vi "Dequeue Message.vi"(8 "Error In":errorcluster, 11 "Message Queue":refnum<queue>) -> (0 "Error Out":errorcluster, 1 "Message Data":variant, 2 "Message":string, 3 "dup Message Queue":refnum<queue>)   [LabVIEW 2017]
uses:
  Desktop/Semestr 8/LabVIEW Advanced/LabVIEW Core 3/Exercises/LabVIEW Core 3/Course Project/support/Message Queue/Message Cluster.ctl
  Desktop/Semestr 8/LabVIEW Advanced/LabVIEW Core 3/Exercises/LabVIEW Core 3/Course Project/support/Message Queue/Message Queue.lvlib
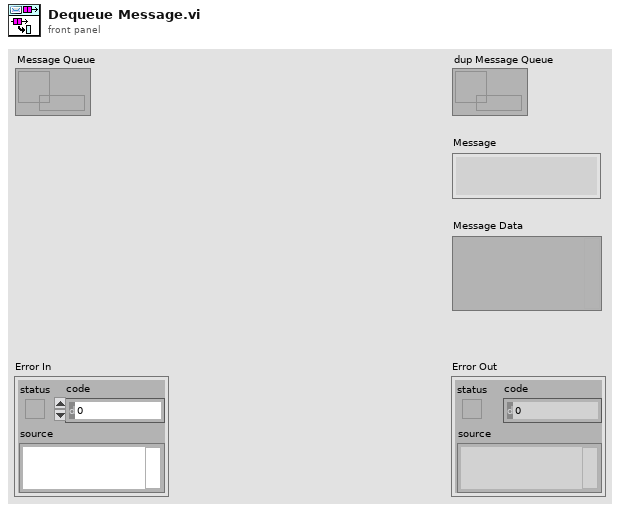
[diagram p1: front panel]
types:
  T1 = typedef "Message Queue.lvlib/Message Cluster.ctl" = cluster{"Message":string, "Message Data":variant}
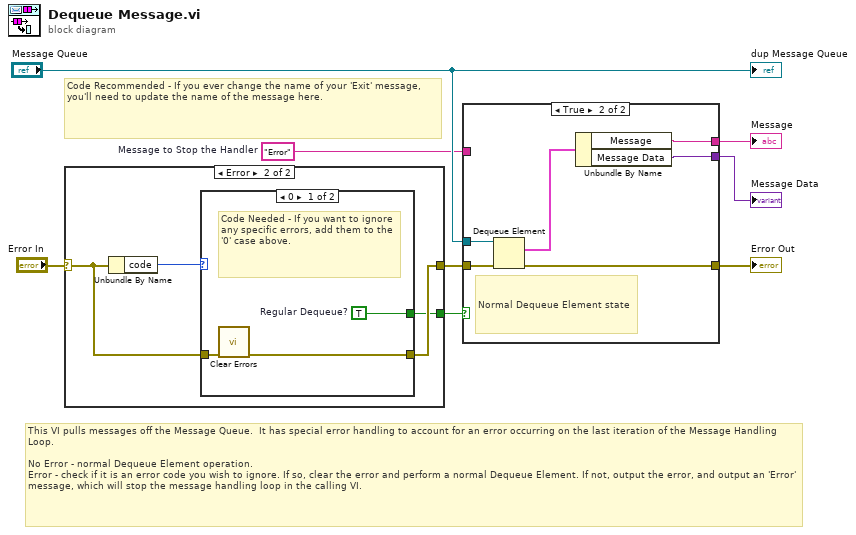
[diagram p0: block diagram]
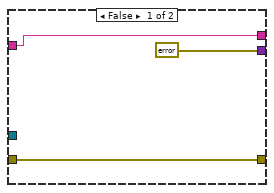
[diagram p2: hidden frame]
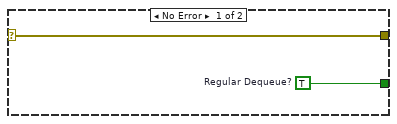
[diagram p3: hidden frame]
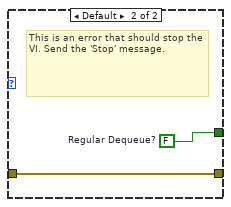
[diagram p4: hidden frame]
diagram:
  w1 = "Error"  # Message to Stop the Handler
  # "Code Recommended - If you ever change the name of your 'Exit' message, you'll need to update the name of the message here."
  # "This VI pulls messages off the Message Queue.  It has special error handling to account for an error occurring on the last iteration of the Message Handling Loop.\n\nNo Error - normal Dequeue Element operation.\nError - check if it is an error code you wish to ignore. If so, clear the error and perform a normal Dequeue Element. If not, output the error, and output an 'Error' message, which will stop the message handling loop in the calling VI."
  n1 = case shown="Error" "Error In" {
    selector: "Error In" -> [w10 w13]
    tunnel: [w10 w12] -> w6
    tunnel: [w9 w11] -> w5
    frame No Error {
      w9 = TRUE  # Regular Dequeue?
    }
    frame Error {
      n2 = Unbundle By Name(w13) -> ("code"=w14:i32)
      n3 = case shown="0" w14 {
        tunnel: [w17 w19] -> w12
        tunnel: w13 -> [w16 w19]
        tunnel: [w15 w18] -> w11
        frame 0 {
          w15 = TRUE  # Regular Dequeue?
          # "Code Needed - If you want to ignore any specific errors, add them to the '0' case above."
          n4 = call <vilib>:"Clear Errors.vi"("error in (no error)"=w16) -> ("error out"=w17:errorcluster)  [unwired: 5 in, 1 out]
        }
        frame Default {
          w18 = FALSE  # Regular Dequeue?
          # "This is an error that should stop the VI. Send the 'Stop' message."
        }
      }
    }
  }
  n5 = case shown="True" w5 {
    tunnel: [w22 w28] -> w7
    tunnel: w6 -> [w22 w27]
    tunnel: "Message Queue" -> [_ w26]
    tunnel: [w21 w24] -> w3
    tunnel: [errorcluster {"status"=FALSE, "code"=0, "source"=""} ("error IO") w23] -> w2
    tunnel: w1 -> [w21 _]
    frame False {
    }
    frame True {
      # "Normal Dequeue Element state"
      n6 = Dequeue Element(queue=w26, error in (no error)=w27) -> (element=w25:T1, error out=w28:errorcluster)  [unwired: 1 in, 2 out]
      n7 = Unbundle By Name(w25) -> ("Message"=w24:string, "Message Data"=w23:variant)
    }
  }
  "Error Out" <- w7
  "Message" <- w3
  "Message Data" <- w2
  "dup Message Queue" <- "Message Queue"
